vi "parse_CMDInput.vi"(8 "error in":errorcluster, 11 "msg in":string) -> (0 "error out":errorcluster, 2 "CMD Input":T1, 3 "msg out":string)   [LabVIEW 2018]
uses:
  std_msgs/subs/parse_float64_scalar.vi
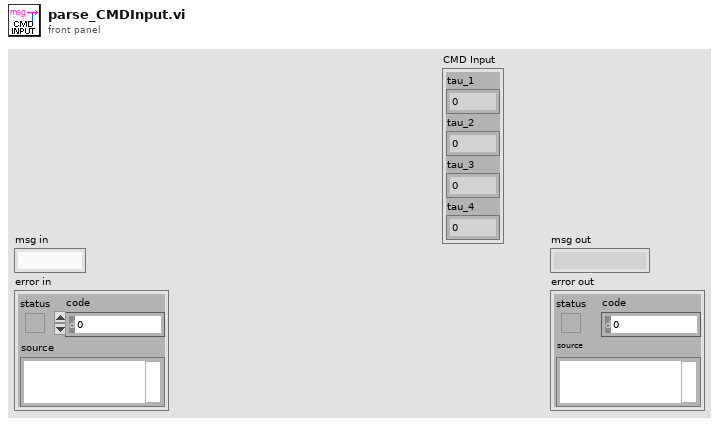
[diagram p1: front panel]
types:
  T1 = cluster{"tau_1":dbl, "tau_2":dbl, "tau_3":dbl, "tau_4":dbl}
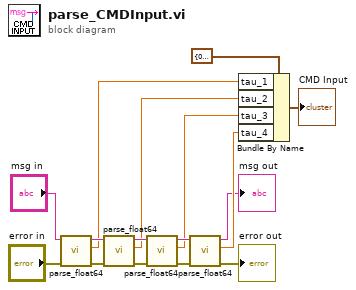
[diagram p0: block diagram]
diagram:
  n1 = call-poly "parse_float64.vi"("error in"="error in", "msg in"="msg in") -> ("error out"=w11:errorcluster, "number"=w8:dbl, "msg out"=w15:string)  [unwired: 3 in]
  n2 = call-poly "parse_float64.vi"("error in"=w11, "msg in"=w15) -> ("error out"=w10:errorcluster, "number"=w7:dbl, "msg out"=w14:string)  [unwired: 3 in]
  n3 = call-poly "parse_float64.vi"("error in"=w10, "msg in"=w14) -> ("error out"=w9:errorcluster, "number"=w6:dbl, "msg out"=w13:string)  [unwired: 3 in]
  n4 = call-poly "parse_float64.vi"("error in"=w9, "msg in"=w13) -> ("error out"=→"error out":errorcluster, "number"=w5:dbl, "msg out"=→"msg out":string)  [unwired: 3 in]
  n5 = Bundle By Name(cluster=T1 {"tau_1"=0.0, "tau_2"=0.0, "tau_3"=0.0, "tau_4"=0.0} ("Input"), "tau_1"=w8, "tau_2"=w7, "tau_3"=w6, "tau_4"=w5) -> (→"CMD Input":T1)
